vi "Simple Open Raw Data File.vi"() -> ()   [LabVIEW 2016]
panel:
  in  "Use Ephys":bool
  out "Waveform Graph":dbl[][](graph)
  in  "Ofset from start (s)":i64
  in  "file path (use dialog)":path=path "C:/Test/2017-07-20/Experiment 013/Raw.bin"
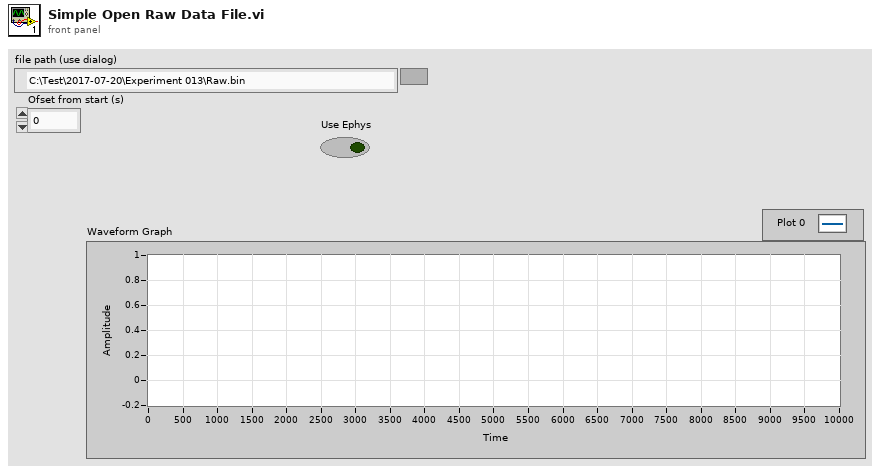
[diagram p1: front panel]
types:
  T1 = enum16{"big-endian, network order", "native, host order", "little-endian"}
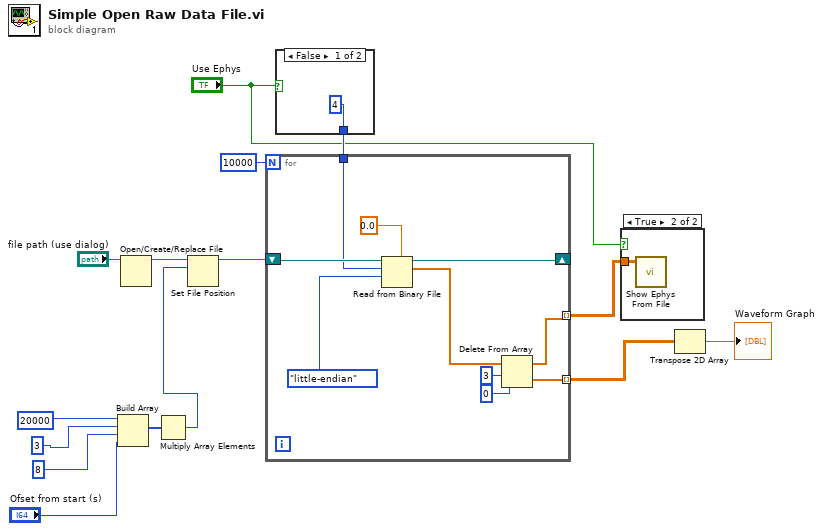
[diagram p0: block diagram]
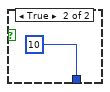
[diagram p3: hidden frame]
diagram:
  n1 = Build Array(i64 20000 ("offset (in bytes) (0)"), i64 3 ("offset (in bytes) (0)"), i64 8 ("offset (in bytes) (0)"), "Ofset from start (s)") -> (w7:i64[])
  n2 = Open/Create/Replace File(file path (use dialog)="file path (use dialog)") -> (refnum out=w13:refnum<file>)  [unwired: 5 in, 2 out]
  n3 = Multiply Array Elements(1:w7) -> (0:w6:i64)
  n4 = Set File Position(offset (in bytes) (0)=w6, refnum=w13) -> (refnum out=w12:refnum<file>)  [unwired: 2 in, 1 out]
  n5 = case shown="False" "Use Ephys" {
    tunnel: [4 ("count (1)") 10 ("count (1)")] -> w3
    frame False {
    }
    frame True {
    }
  }
  n6 = for {
    N: 10000 -> [_]
    shift-right: [w26] -> _
    shift-left: w12 -> [w27]
    tunnel: [w18] -> w5 mode=indexing
    tunnel: w3 -> [w23]
    tunnel: [w19] -> w2 mode=indexing
    n7 = Read from Binary File(5:0.0, 9:T1."little-endian" ("byte order (0:big-endian, network order)"), 10:w23, 11:w27) -> (2:w22:dbl[], 3:w26:refnum<file>)  [unwired: 2 in, 2 out]
    n8 = Delete From Array(array=w22, length=3, index=0) -> (deleted portion=w18:dbl[], array with subset deleted=w19:dbl[])
  }
  n9 = case shown="True" "Use Ephys" {
    tunnel: w2 -> [_ w28]
    frame False {
    }
    frame True {
      n10 = call "Show Ephys From File.vi"("Array"=w28) -> ()  [unwired: 11 in]
    }
  }
  n11 = Transpose 2D Array(2D array=w5) -> (transposed array=→"Waveform Graph":dbl[][])
